vi "motorControl.vi"() -> ()   [LabVIEW 2018]
uses:
  driveStateEnum.ctl
  conversionTypeEnum.ctl
  <vilib>/Rock Robotics/WPI/ThirdParty/Phoenix-LabVIEW/Motor Controller/Controls/CTRE_Phoenix_MotorControl_ControlMode.ctl
  <vilib>/Rock Robotics/WPI/Utilities/WPI_GetSetVariantRefNum.vi
  <vilib>/Rock Robotics/WPI/ThirdParty/Phoenix-LabVIEW/Motor Controller/Get/CTRE_Phoenix_MotorController_GetSelectedSensorData.vi
panel:
  out "Encoder Position (Inches)":dbl
  out "Encoder Position (Raw Units)":i32
  in  "Motion Magic Objective (Inches)":dbl format="%#_6f"
  out "Motion Magic Objective (Raw Units)":dbl
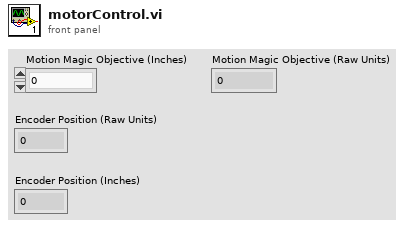
[diagram p1: front panel]
types:
  T1 = typedef "WPI_JoystickDevRef.ctl" = cluster{"Device":T2}
  T2 = typedef "WPI_JoystickDeviceEnum.ctl" = enum16{"USB 0", "USB 1", "USB 2", "USB 3", "USB 4", "USB 5"}
  T3 = typedef "WPI_MotorControlDeviceRef.ctl" = cluster{"DeviceStatus":errorcluster, "Type":T4, "PWM":cluster{"PWM Channel":T5, "DeadBand":T6}, "CAN":cluster{"Device Number":u8, "SetOutput VI Ref":variant, "GetOutput VI Ref":variant, "Enable VI Ref":variant, "Disable VI Ref":variant, "Data":variant}, "Invert":bool, "DIO PWM":cluster{"PWM \"Enable\" Channel":T5, "DIOChannel":T7, "PWM Rate":dbl}}
  T4 = typedef "WPI_MotorControlType.ctl" = enum16{"PWM", "CAN", "DIO PWM"}
  T5 = typedef "FPGA_DIOPWMChannel.ctl" = enum8{"PWM 0", "PWM 1", "PWM 2", "PWM 3", "PWM 4", "PWM 5", "PWM 6", "PWM 7", "PWM 8", "PWM 9", "PWM MXP 0", "PWM MXP 1", "PWM MXP 2", "PWM MXP 3", "PWM MXP 4", "PWM MXP 5", "PWM MXP 6", "PWM MXP 7", "PWM MXP 8", "PWM MXP 9", "Invalid"}
  T6 = typedef "WPI_PWMDeadband.ctl" = cluster{"Name":string, "maxPositivePwm":i32, "minPositivePwm":i32, "centerPwm":i32, "maxNegativePwm":i32, "minNegativePwm":i32, "angularRange":u16}
  T7 = typedef "FPGA_DIOChannel.ctl" = enum8{"DIO 0", "DIO 1", "DIO 2", "DIO 3", "DIO 4", "DIO 5", "DIO 6", "DIO 7", "DIO 8", "DIO 9", "DIO MXP 0", "DIO MXP 1", "DIO MXP 2", "DIO MXP 3", "DIO MXP 4", "DIO MXP 5", "DIO MXP 6", "DIO MXP 7", "DIO MXP 8", "DIO MXP 9", "DIO MXP 10", "DIO MXP 11", "DIO MXP 12", "DIO MXP 13", "DIO MXP 14", "DIO MXP 15", "SPI Port CS1", "SPI Port CS2", "SPI Port CS3", "SPI Port MISO", "SPI Port MOSI", "Invalid"}
  T8 = typedef "conversionTypeEnum.ctl" = enum16{"Sensor Units -> Inches", "Inches -> Sensor Units"}
  T9 = typedef "driveStateEnum.ctl" = enum16{"Manual", "Motion Magic", "Reset Encoders"}
  T10 = typedef "CTRE_Phoenix_MotorControl_ControlMode.ctl" = u16
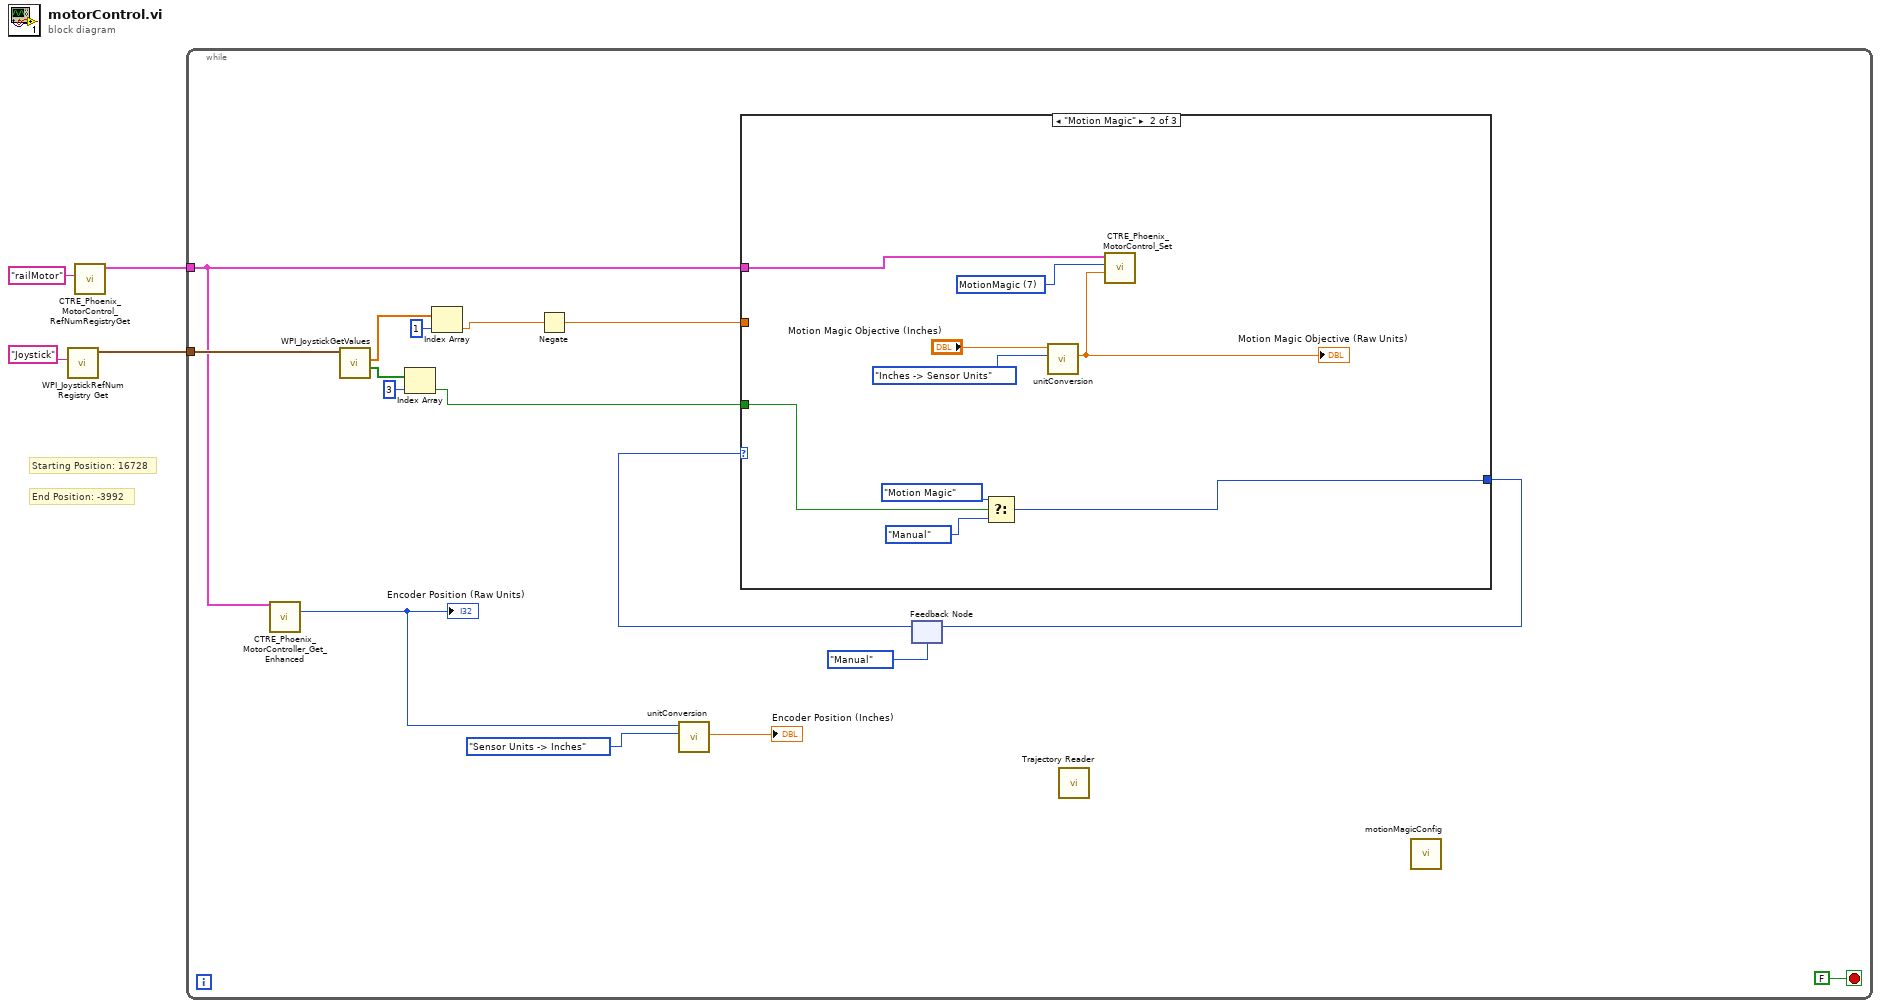
[diagram p0: block diagram]
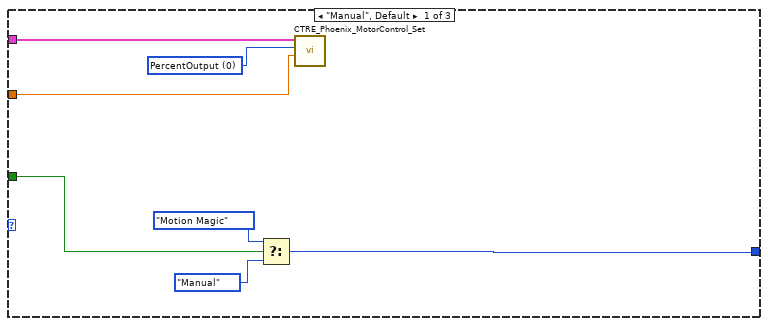
[diagram p2: hidden frame]
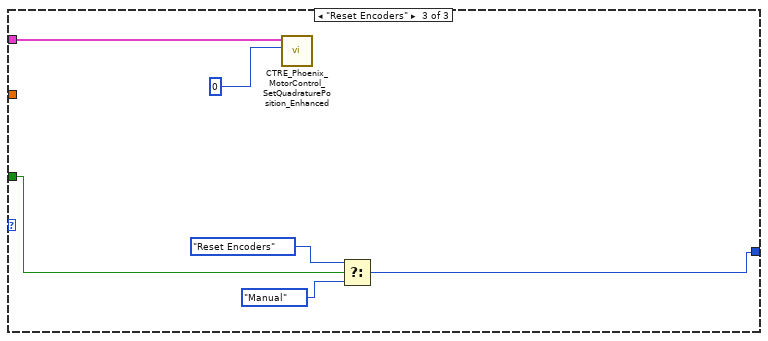
[diagram p3: hidden frame]
diagram:
  # "End Position: -3992"
  # "Starting Position: 16728"
  n1 = call <vilib>:"WPI_JoystickRefNum Registry Get.vi"("refnum name"="Joystick") -> ("JoystickDevRef"=w3:T1)  [unwired: 9 in, 1 out]
  n2 = call <vilib>:"CTRE_Phoenix_MotorControl_RefNumRegistryGet.vi"("refnum name"="railMotor") -> ("PhoenixMotorControlDevRef"=w1:T3)  [unwired: 9 in, 1 out]
  n3 = while {
    tunnel: w3 -> [w17]
    tunnel: w1 -> [w5]
    stop <- FALSE stop-if-true
    n4 = call-poly <vilib>:"CTRE_Phoenix_MotorController_Get_Enhanced.vi"("PhoenixMotorControlDevRef"=w5) -> ("Position (Raw Sensor Units)"=w9:i32)  [unwired: 11 in, 3 out]
    "Encoder Position (Raw Units)" <- w9
    n5 = call <vilib>:"WPI_JoystickGetValues.vi"("JoystickDevRef"=w17) -> ("Buttons"=w16:bool[], "Axes"=w13:dbl[])  [unwired: 6 in, 3 out]
    n6 = Index Array(array=w16, index=3) -> (element=w10:bool)
    n7 = Index Array(array=w13, index=1) -> (element=w11:dbl)
    n8 = Negate(x=w11) -> (-x=w6:dbl)
    n9 = call "unitConversion.vi"("Conversion Type"=conversionTypeEnum."Sensor Units -> Inches", "Units to Convert"=w9) -> ("Conversion Result"=→"Encoder Position (Inches)":dbl)  [unwired: 9 in]
    n10 = feedback #1(driveStateEnum."Manual") -> (w18:T9)
    n11 = case shown="\"Motion Magic\"" w18 {
      tunnel: w10 -> [w27 w36 w39]
      tunnel: [w24 w35 w40] -> w14
      tunnel: w5 -> [w23 w33 w38]
      tunnel: w6 -> [w21 _ _]
      frame "Manual", Default {
        w22 = T10 0 items=["PercentOutput"=0, "Position"=1, "Velocity"=2, "Current"=3, "Follower"=5, "MotionProfile"=6, "MotionMagic"=7, "MotionProfileArc"=10, "Disabled"=15] ("Control Mode")
        n12 = Select(t=driveStateEnum."Motion Magic", s=w27, f=driveStateEnum."Manual") -> (s? t:f=w24:T9)
        n13 = call <vilib>:"CTRE_Phoenix_MotorControl_Set.vi"("Output"=w21, "Control Mode"=w22, "PhoenixMotorControlDevRef"=w23) -> ()  [unwired: 7 in, 2 out]
      }
      frame "Motion Magic" {
        w34 = T10 7 items=["PercentOutput"=0, "Position"=1, "Velocity"=2, "Current"=3, "Follower"=5, "MotionProfile"=6, "MotionMagic"=7, "MotionProfileArc"=10, "Disabled"=15] ("Control Mode")
        n14 = Select(t=driveStateEnum."Motion Magic", s=w36, f=driveStateEnum."Manual") -> (s? t:f=w35:T9)
        n15 = call "unitConversion.vi"("Conversion Type"=conversionTypeEnum."Inches -> Sensor Units", "Units to Convert"="Motion Magic Objective (Inches)") -> ("Conversion Result"=w28:dbl)  [unwired: 9 in]
        "Motion Magic Objective (Raw Units)" <- w28
        n16 = call <vilib>:"CTRE_Phoenix_MotorControl_Set.vi"("Output"=w28, "Control Mode"=w34, "PhoenixMotorControlDevRef"=w33) -> ()  [unwired: 7 in, 2 out]
      }
      frame "Reset Encoders" {
        n17 = call <vilib>:"CTRE_Phoenix_MotorControl_SetQuadraturePosition_Enhanced.vi"("New Position"=0, "PhoenixMotorControlDevRef"=w38) -> ()  [unwired: 8 in, 2 out]
        n18 = Select(t=driveStateEnum."Reset Encoders", s=w39, f=driveStateEnum."Manual") -> (s? t:f=w40:T9)
      }
    }
    n19 = feedback-in #1(w14) -> ()
    n20 = call "Trajectory Reader.vi"() -> ()  [unwired: 12 in]
    n21 = call "motionMagicConfig.vi"() -> ()  [unwired: 12 in]
  }
